vi "Asynchronous Process.vi"(11 "Process":i32 format="Process Number: %.0f") -> ()   [LabVIEW 2015]
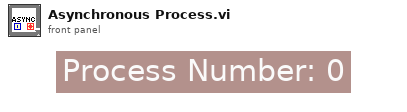
[diagram p1: front panel]
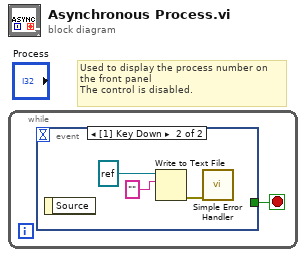
[diagram p0: block diagram]
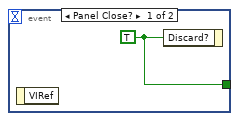
[diagram p2: hidden frame]
diagram:
  # "Used to display the process number on\nthe front panel\nThe control is disabled."
  n1 = while {
    stop <- w1 stop-if-true
    n2 = event shown="[1] Key Down" {
      selector: _ -> [_ _]
      dyn-events: _ -> [_ _]
      timeout: _ -> [_ _]
      tunnel: [w2 _] -> w1
      event Panel Close? {
        w2 = TRUE ("Discard?")
        n3 = event-data() -> ()  [unwired: 1 in, 1 out]
        n4 = event-data("Discard?"=w2) -> ()  [unwired: 1 in, 1 out]
      }
      event Key Down {
        n5 = event-data() -> ()  [unwired: 1 in, 1 out]
        n6 = Write to Text File(file (use dialog)=refnum<file> refnum ("refnum out"), text="") -> (error out=w3:errorcluster)  [unwired: 2 in, 2 out]
        n7 = call <vilib>:"Simple Error Handler.vi"("error in (no error)"=w3) -> ()  [unwired: 4 in, 5 out]
      }
    }
  }
